vi "save_motor_positions_to_log_file.vi"(6 "Save Time (s)":i32, 8 "error in":errorcluster, 10 "Manipulator Pos (Steps)":i32[](array[numeric]), 11 "file path":path) -> (0 "error out":errorcluster, 3 "path":path)   [LabVIEW 2018]
uses:
  Save_Time_Global.vi
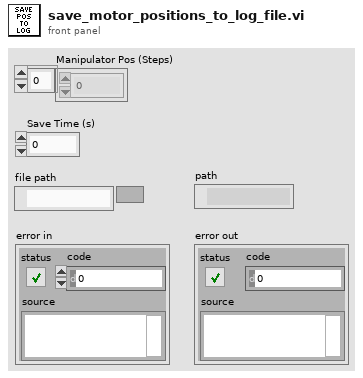
[diagram p1: front panel]
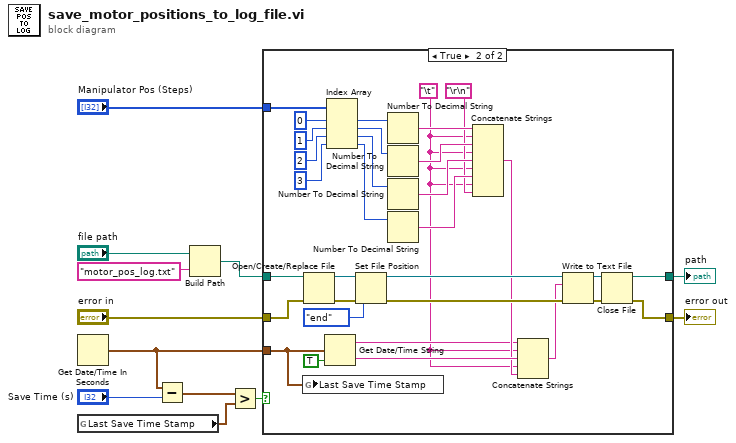
[diagram p0: block diagram]
diagram:
  n1 = Get Date/Time In Seconds() -> (seconds since 1Jan1904=w5:timestamp)
  n2 = global read "Save_Time_Global.vi" "Last Save Time Stamp"() -> (w6:timestamp)
  n3 = Subtract(x=w5, y="Save Time (s)") -> (x-y=w7:timestamp)
  n4 = Build Path(base path="file path", name or relative path="motor_pos_log.txt") -> (appended path=w2:path)
  n5 = Greater?(x=w7, y=w6) -> (0:w4:bool)
  n6 = case shown="True" w4 {
    tunnel: "Manipulator Pos (Steps)" -> [_ w46]
    tunnel: w2 -> [w14 w27]
    tunnel: "error in" -> [w13 w26]
    tunnel: [w13 w23] -> w10
    tunnel: [w14 w22] -> w9
    tunnel: w5 -> [_ w20]
    frame False {
    }
    frame True {
      w15 = "\t"
      n7 = global write "Save_Time_Global.vi" "Last Save Time Stamp"(w20) -> ()
      n8 = Open/Create/Replace File(file path (use dialog)=w27, error in=w26) -> (refnum out=w33:refnum<file>, error out=w30:errorcluster)  [unwired: 4 in, 1 out]
      n9 = Get Date/Time String(seconds (now)=w20, want seconds? (F)=TRUE) -> (date string=w16:string, time string=w19:string)  [unwired: 1 in]
      n10 = Index Array(array=w46, index #1=0 ("index"), index #2=1 ("index"), index #3=2 ("index"), index #4=3 ("index")) -> (element #1=w41:i32, element #2=w40:i32, element #3=w39:i32, element #4=w38:i32)
      n11 = Set File Position(refnum=w33, from (0:start)=enum16{"start", "end", "current"}."end", error in=w30) -> (refnum out=w32:refnum<file>, error out=w29:errorcluster)  [unwired: 1 in]
      n12 = Number To Decimal String(number=w41) -> (decimal integer string=w37:string)  [unwired: 1 in]
      n13 = Number To Decimal String(number=w40) -> (decimal integer string=w36:string)  [unwired: 1 in]
      n14 = Number To Decimal String(number=w39) -> (decimal integer string=w35:string)  [unwired: 1 in]
      n15 = Number To Decimal String(number=w38) -> (decimal integer string=w34:string)  [unwired: 1 in]
      n16 = Concatenate Strings(w37, w15, w36, w15, w35, w15, w34, w15, "\r\n") -> (w18:string)
      n17 = Concatenate Strings(w16, w15, w19, w15, w18) -> (w17:string)
      n18 = Write to Text File(file (use dialog)=w32, text=w17, error in=w29) -> (refnum out=w31:refnum<file>, error out=w28:errorcluster)  [unwired: 1 in, 1 out]
      n19 = Close File(refnum=w31, error in=w28) -> (path=w22:path, error out=w23:errorcluster)
    }
  }
  "error out" <- w10
  "path" <- w9
